vi "Evaluate In Range Trigger.vi"(8 "error in (no error)":errorcluster, 10 "Trigger Data":dbl[](array[numeric]), 11 "In Range Trigger in":refnum<class "In Range Trigger.lvclass">) -> (0 "error out":errorcluster, 2 "Trigger":bool, 3 "In Range Trigger out":refnum<class "In Range Trigger.lvclass">)   [LabVIEW 2015, in "Waveform Data Logger Engine.lvlib" / "In Range Trigger.lvclass"]
uses:
  In Range Trigger.lvclass
  In Range Trigger.lvclass/In Range Trigger.ctl
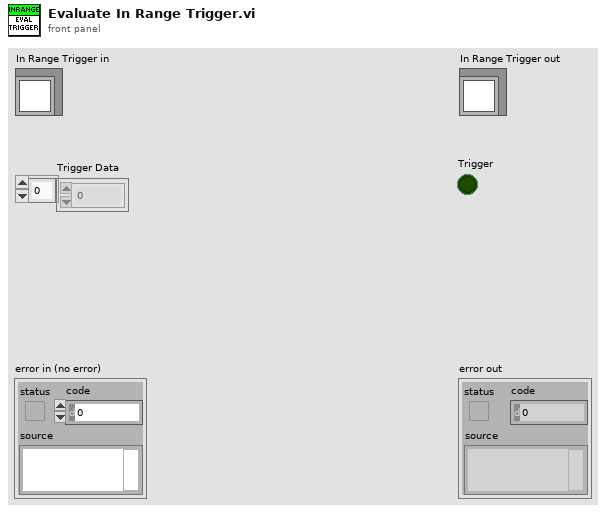
[diagram p1: front panel]
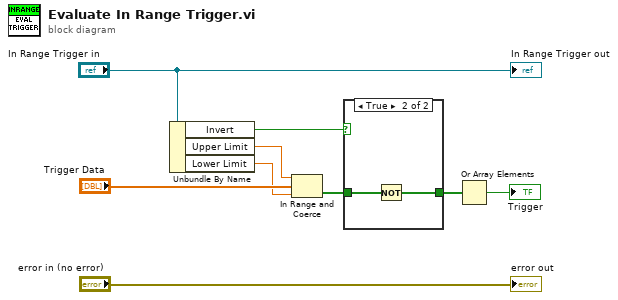
[diagram p0: block diagram]
diagram:
  n1 = Unbundle By Name("In Range Trigger in") -> ("Invert"=w4:bool, "Upper Limit"=w6:dbl, "Lower Limit"=w5:dbl)
  n2 = In Range and Coerce(upper limit=w6, x="Trigger Data", lower limit=w5) -> (In Range?=w3:bool[])  [unwired: 1 out]
  n3 = case shown="True" w4 {
    tunnel: [w10 w12] -> w2
    tunnel: w3 -> [w10 w11]
    frame False {
    }
    frame True {
      n4 = Not(x=w11) -> (.not. x?=w12:bool[])
    }
  }
  n5 = Or Array Elements(Boolean array=w2) -> (logical OR=→"Trigger":bool)
  "error out" <- "error in (no error)"
  "In Range Trigger out" <- "In Range Trigger in"
